vi "Verify LEUI Binary Blinking.vi"(0 "GEA2 Reference In":refnum<k24>, 1 "Standalone":bool, 2 "Initial Timeout (s)":dbl, 5 "Numeric":u8, 7 "Retry Count":i32, 9 "Max Blink Rate (sec)":dbl, 11 "Error In":errorcluster, 12 "Ignore Brightness":bool) -> (4 "GEA2 Reference Out":refnum<k24>, 6 "Pass/Fail?":bool, 10 "Report Text":string, 14 "Blink Times (s)":dbl[](array[numeric]), 15 "Error Out":errorcluster)   [LabVIEW 2016, in "TLMB.lvlib"]
uses:
  Projects/TLMB.lvlib
  Q:/Common/DLLs/GEA3/GeaCommunication.dll
  Common/DLLs/GEA3/GeaCommunication.dll
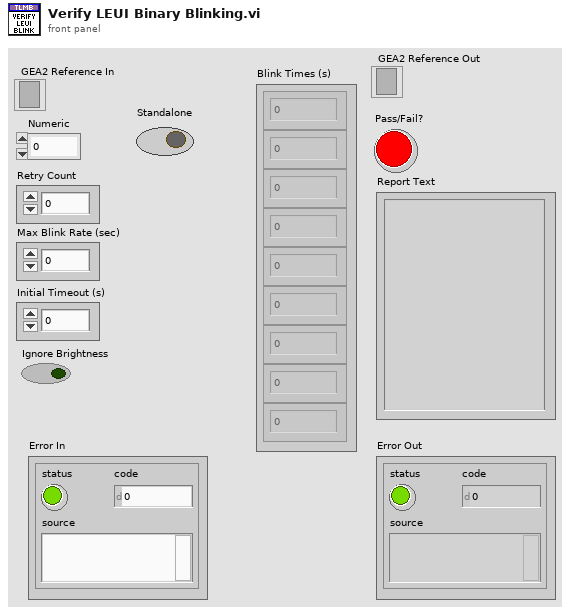
[diagram p1: front panel]
types:
  T1 = typedef "TLMB.lvlib/LEUI_LEDs.ctl" = cluster{"Pause (Z401)":bool, "Lid Locked (Z402)":bool, "LED1 (Z407)":bool, "LED2 (Z406)":bool, "LED3 (Z405)":bool, "LED4 (Z404)":bool, "LED5 (Z403)":bool, "LED6 (Z409)":bool, "Option 1 (Z408)":bool, "Option 2 (Z410)":bool}
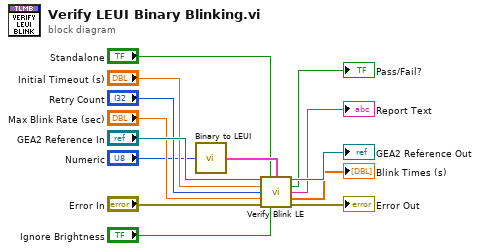
[diagram p0: block diagram]
diagram:
  n1 = call "Binary to LEUI.vi"("Numeric"="Numeric") -> ("Blinking LED"=w14:T1)  [unwired: 14 in]
  n2 = call "Verify Blink LE.vi"("GEA2 Reference In"="GEA2 Reference In", "Standalone"="Standalone", "Blinking LED"=w14, "Initial Timeout (s)"="Initial Timeout (s)", "Retry Count"="Retry Count", "Max Blink Rate (sec)"="Max Blink Rate (sec)", "Error In"="Error In", "Ignore Brightness"="Ignore Brightness") -> ("GEA2 Reference Out"=→"GEA2 Reference Out":refnum<k24>, "Pass/Fail?"=→"Pass/Fail?":bool, "Report Text"=→"Report Text":string, "Blink Times (s)"=→"Blink Times (s)":dbl[], "Error Out"=→"Error Out":errorcluster)  [unwired: 3 in]
